vi "to string.vi"(8 "error in":errorcluster, 11 "user tag bus module configuration In":refnum<class "TEST CONFIGURATION.lvclass">) -> (0 "error out":errorcluster, 1 "data":string, 2 "version":string, 3 "user tag bus module configuration Out":refnum<class "TEST CONFIGURATION.lvclass">)   [LabVIEW 2013, in "configuration tests.lvlib" / "TEST CONFIGURATION.lvclass"]
doc: "Provides an interface for saving a module configuration to a file or other serialized data source. It is recommended that all children of this class store data in two sets--data required for its own initialization, and any data required for parent initialization--and that each implementation uses the <b>Call Parent Method</b> primitive to serialize parent information."
uses:
  TEST CONFIGURATION.lvclass
  <vilib>/NI/Tag Bus Module Framework/module configuration/TBM module configuration.lvclass
  TEST CONFIGURATION.lvclass/TEST CONFIGURATION.ctl
  current version.vi
  <vilib>/NI/Configuration Framework/serializable configuration/NISE_CEF_serializable configuration.lvclass
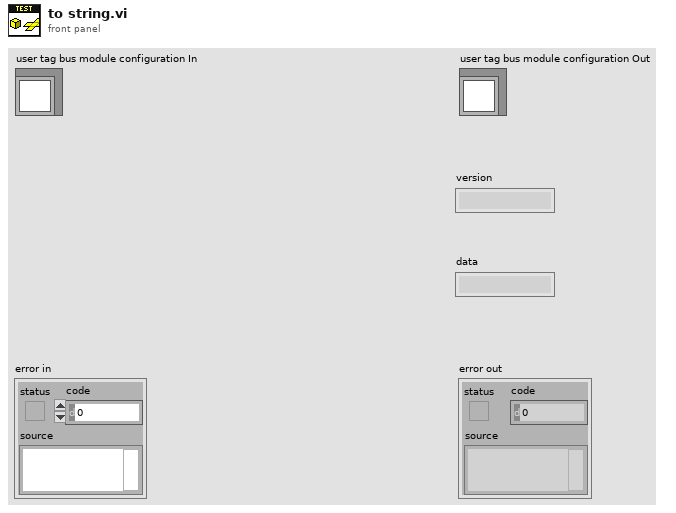
[diagram p1: front panel]
types:
  T1 = typedef "configuration tests.lvlib/TEST CONFIGURATION.lvclass/state module configuration.ctl" = cluster{"fixed input":refnum<class "TBM channel.lvclass">, "fixed output":refnum<class "TBM channel.lvclass">, "initial state":u8}
  T2 = typedef "configuration tests.lvlib/TEST CONFIGURATION.lvclass/control module configuration.ctl" = cluster{"name":string, "setpoint":refnum<class "TBM channel.lvclass">, "process variable":refnum<class "TBM channel.lvclass">, "output":refnum<class "TBM channel.lvclass">, "gains":T3, "output range":cluster{"output high":dbl, "output low":dbl}}
  T3 = typedef "configuration tests.lvlib/TEST CONFIGURATION.lvclass/gains.ctl" = cluster{"Kp":dbl, "Ki":dbl, "Kd":dbl}
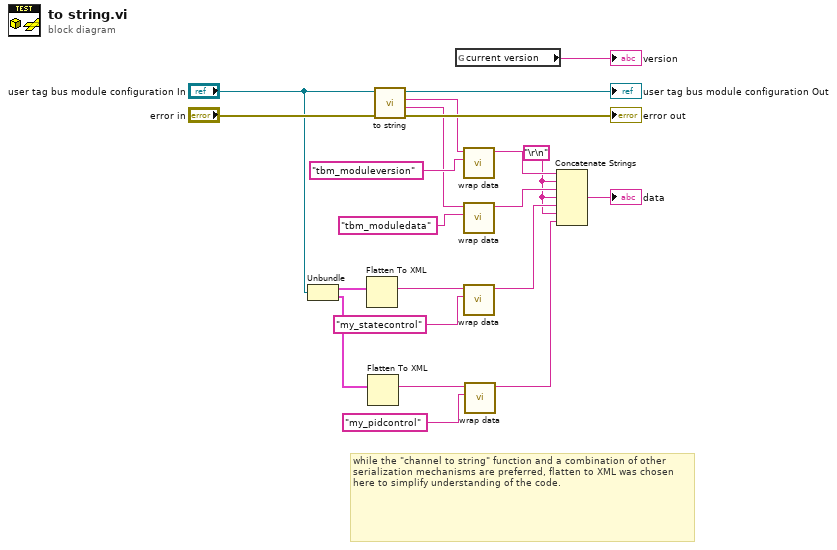
[diagram p0: block diagram]
diagram:
  w1 = "\r\n"
  # "while the \"channel to string\" function and a combination of other serialization mechanisms are preferred, flatten to XML was chosen here to simplify understanding of the code."
  n1 = Unbundle("user tag bus module configuration In") -> (w4:T1, w3:T2[])
  n2 = Flatten To XML(anything=w4) -> (xml string=w9:string)
  n3 = Flatten To XML(anything=w3) -> (xml string=w5:string)
  n4 = call-parent "to string.vi"("error in"="error in", "module configuration in"="user tag bus module configuration In") -> ("error out"=→"error out":errorcluster, "data"=w12:string, "version"=w13:string, "module configuration out"=→"user tag bus module configuration Out":refnum<class "TEST CONFIGURATION.lvclass">)  [unwired: 6 in]
  n5 = global read "current version.vi" "current version"() -> (→"version":string)
  n6 = call <vilib>:"wrap data.vi"("identifier"="tbm_moduleversion" ("additional identifier"), "data to wrap"=w13) -> ("wrapped data"=w15:string)  [unwired: 9 in]
  n7 = call <vilib>:"wrap data.vi"("identifier"="tbm_moduledata" ("additional identifier"), "data to wrap"=w12) -> ("wrapped data"=w14:string)  [unwired: 9 in]
  n8 = call <vilib>:"wrap data.vi"("identifier"="my_statecontrol" ("additional identifier"), "data to wrap"=w9) -> ("wrapped data"=w8:string)  [unwired: 9 in]
  n9 = call <vilib>:"wrap data.vi"("identifier"="my_pidcontrol" ("additional identifier"), "data to wrap"=w5) -> ("wrapped data"=w2:string)  [unwired: 9 in]
  n10 = Concatenate Strings(w15, w1, w14, w1, w8, w1, w2) -> (→"data":string)
